vi "Ping.vi"(8 "Error In":errorcluster, 11 "CS++RTRootActor in":refnum<class "CS++RTRootActor.lvclass">) -> (0 "Error Out":errorcluster, 3 "CS++RTRootActor out":refnum<class "CS++RTRootActor.lvclass">)   [LabVIEW 2015]
doc: "Increment attribute and publish to SV."
uses:
  CS++RTRootActor.lvclass
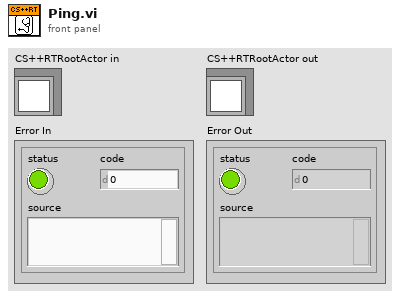
[diagram p1: front panel]
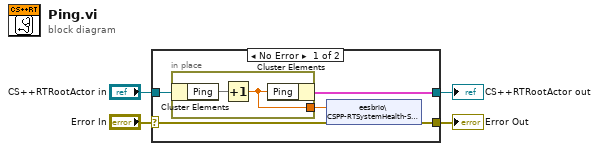
[diagram p0: block diagram]
diagram:
  n1 = case shown="No Error" "Error In" {
    selector: "Error In" -> [w6 w13]
    tunnel: [w5 w13] -> w3
    tunnel: [w8 w12] -> w1
    tunnel: "CS++RTRootActor in" -> [w9 w12]
    frame No Error {
      n2 = in-place {
        in-place-border: [w10] -> w7
        n3 = in-place-cluster #1(w9) -> ("Ping"=w11)
        n4 = Increment(x=w11) -> (x+1=w10:dbl)
        n5 = in-place-cluster #1("Ping"=w10) -> (w8:cluster{})
      }
      n6 = shared-variable "eesbrio\\CSPP-RTSystemHealth-SV.lvlib\\LNA Ping"(w7, error in=w6) -> (error out=w5:errorcluster)
    }
    frame Error {
    }
  }
  "Error Out" <- w3
  "CS++RTRootActor out" <- w1
